vi "UpdateConditions.vi"(6 "ConditionType":T3, 7 "data group":string, 8 "error in (no error)":errorcluster, 9 "OpState":i32, 10 "conditions":T1[](array[typedef]), 11 "operating states in":variant) -> (0 "error out":errorcluster, 3 "operating states out":variant)   [LabVIEW 2017, in "OpState.lvlib"]
uses:
  <vilib>/addons/InsightCM/Devices/Shared/Common/OpState/OpState.lvlib
  <vilib>/addons/InsightCM/Devices/Shared/Common/OpState/controls/ConditionType.ctl
  <vilib>/addons/InsightCM/Devices/Shared/Common/Trigger/controls/TriggerCondition.ctl
  <vilib>/addons/InsightCM/MessageBus/Base/controls/Condition.ctl
  <vilib>/addons/InsightCM/Devices/Shared/Common/OpState/controls/TriggerOperatingState.ctl
  <vilib>/addons/InsightCM/MessageBus/Base/controls/KeyValuePair.ctl
  <vilib>/addons/InsightCM/Devices/Shared/Common/Trigger/Trigger.lvlib
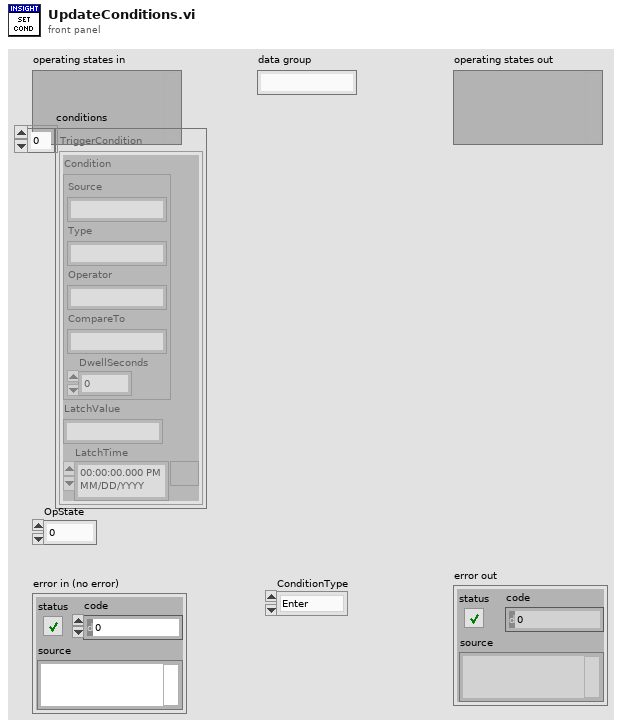
[diagram p1: front panel]
types:
  T1 = typedef "Trigger.lvlib/TriggerCondition.ctl" = cluster{"Condition":T2, "LatchValue":string, "LatchTime":timestamp}
  T2 = typedef "Condition.ctl" = cluster{"Source":string, "Type":string, "Operator":string, "CompareTo":string, "DwellSeconds":dbl}
  T3 = typedef "OpState.lvlib/ConditionType.ctl" = enum16{"Enter", "Exit"}
  T4 = typedef "OpState.lvlib/TriggerOperatingState.ctl" = cluster{"Id":string, "Name":string, "Properties":T5[], "EnterExpression":string, "EnterConditions":T1[], "ExitExpression":string, "ExitConditions":T1[]}
  T5 = typedef "KeyValuePair.ctl" = cluster{"Key":string, "Value":string}
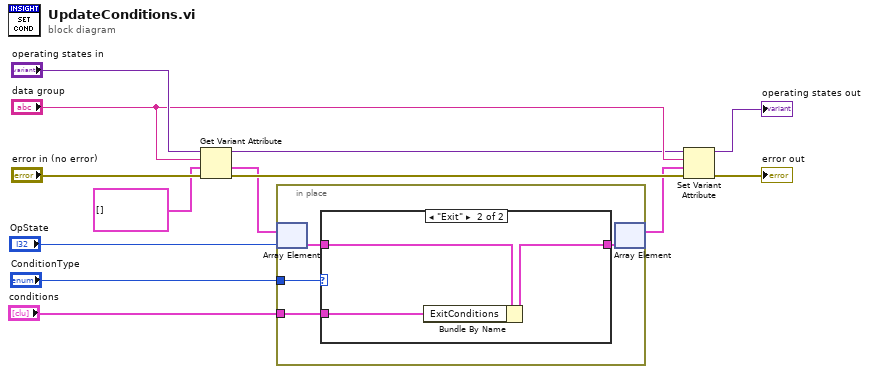
[diagram p0: block diagram]
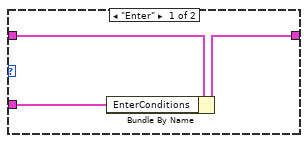
[diagram p2: hidden frame]
diagram:
  n1 = Get Variant Attribute(Variant="operating states in", name="data group", default value (empty Variant)=T4[] [] ("OperatingStates"), error in="error in (no error)") -> (duplicate Variant=w3:variant, value=w7:T4[], error out=w9:errorcluster)  [unwired: 1 out]
  n2 = in-place {
    in-place-border: "ConditionType" -> [w17]
    in-place-border: "conditions" -> [w14]
    n3 = in-place-array #1(w7, "OpState") -> (w16:T4)
    n4 = case shown="\"Exit\"" w17 {
      tunnel: w16 -> [w20 w23]
      tunnel: [w19 w22] -> w15
      tunnel: w14 -> [w18 w21]
      frame "Enter" {
        n5 = Bundle By Name(cluster=w20, "EnterConditions"=w18) -> (w19:T4)
      }
      frame "Exit" {
        n6 = Bundle By Name(cluster=w23, "ExitConditions"=w21) -> (w22:T4)
      }
    }
    n7 = in-place-array #1(w15) -> (w5:T4[])  [unwired: 1 out]
  }
  n8 = Set Variant Attribute(Variant=w3, name="data group", value=w5, error in=w9) -> (Variant out=→"operating states out":variant, error out=→"error out":errorcluster)  [unwired: 1 out]
